vi "Send Command.vi"(0 "connection ID":refnum<k5>, 5 "Command":u8=3 format="%.0x", 7 "Message":string, 9 "Timeout (15s)":dbl=15.0, 11 "error in (no error)":errorcluster) -> (4 "connection ID out":refnum<k5>, 15 "error out":errorcluster)   [LabVIEW 2014, in "hse-db.lvlib" / "MySQL (TCP).lvlib"]
uses:
  MySQL (TCP).lvlib
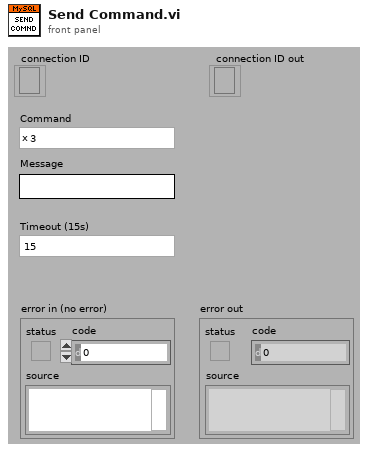
[diagram p1: front panel]
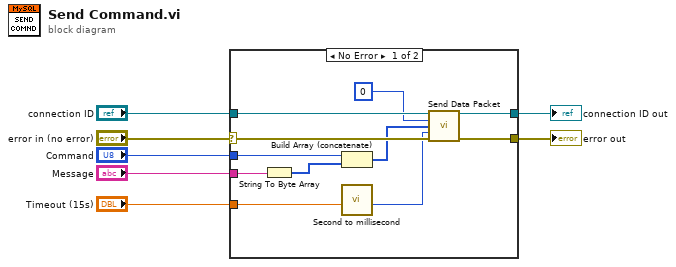
[diagram p0: block diagram]
diagram:
  n1 = case shown="No Error" "error in (no error)" {
    selector: "error in (no error)" -> [w18 w20]
    tunnel: [w17 w20] -> w6
    tunnel: [w15 w19] -> w5
    tunnel: "connection ID" -> [w16 w19]
    tunnel: "Message" -> [w14 _]
    tunnel: "Command" -> [w10 _]
    tunnel: "Timeout (15s)" -> [w9 _]
    frame No Error {
      n2 = String To Byte Array(string=w14) -> (unsigned byte array=w13:u8[])
      n3 = Build Array (concatenate)(w10, w13) -> (w12:u8[])
      n4 = call "Second to millisecond.vi"("Timeout"=w9) -> ("Timeout (ms)"=w8:i32)  [unwired: 10 in]
      n5 = call "Send Data Packet.vi"("connection ID"=w16, "Packet #"=u8 0, "TCP/IP Data"=w12, "Timeout (15000ms)"=w8, "error in"=w18) -> ("connection ID out"=w15:refnum<k5>, "error out"=w17:errorcluster)  [unwired: 9 in]
    }
    frame Error {
    }
  }
  "error out" <- w6
  "connection ID out" <- w5
